vi "Write Tab-Delimited File.vi"() -> ()   [LabVIEW 2023]
doc: "Converts an array of data to a row of tab-separated columns, prepends the timestamp column, and terminates each row with the end of line character."
panel:
  out "Current Data":dbl[](graph)
  # "Overview: Demonstrates the use of the File I/O functions to write data to a tab-delimited text file.\nInstructions:\n1. Run this VI, which generates 5 sets of random data.\n2. Drag the [LabVIEW Data]\\Example Tab-Delimited File.txt file into a spreadsheet application like Microsoft Excel. The data in the file should be automatically populated in the spreadsheet.\n3. Close the spreadsheet application.\n4. Open Read Tab-Delimited File.vi and follow the instructions on its front panel to see an example of reading tab-delimited data in LabVIEW."
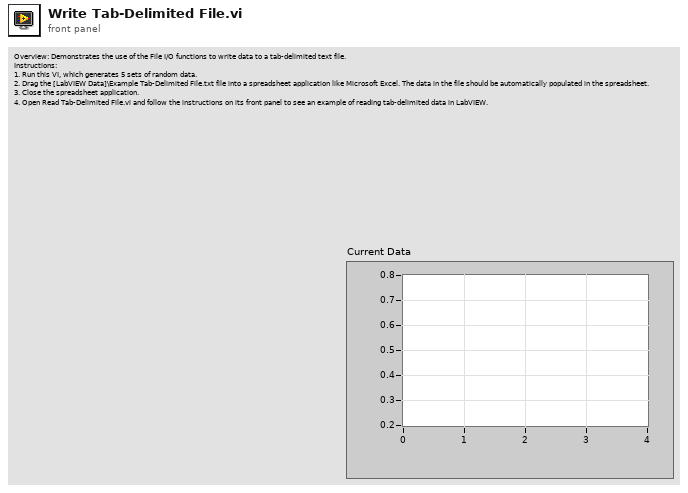
[diagram p1: front panel]
types:
  T1 = enum16{"open", "replace", "create", "open or create", "replace or create", "replace or create with confirmation"}
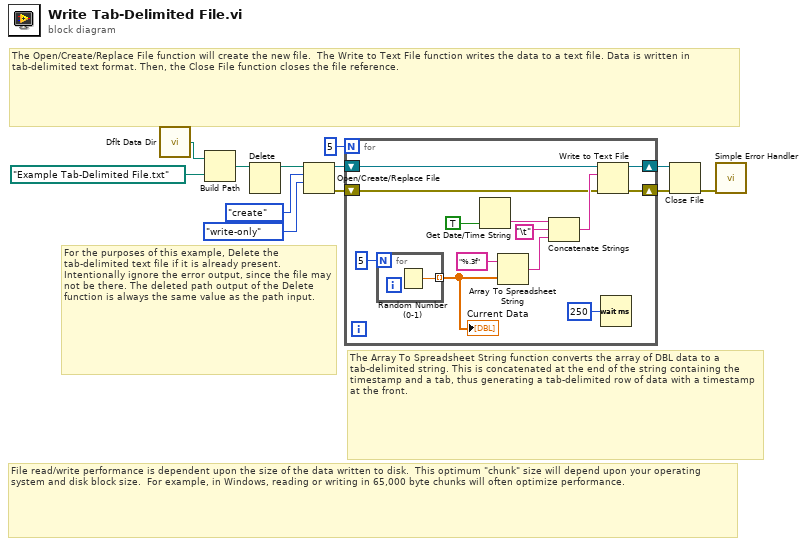
[diagram p0: block diagram]
diagram:
  # "File read/write performance is dependent upon the size of the data written to disk.  This optimum \"chunk\" size will depend upon your operating system and disk block size.  For example, in Windows, reading or writing in 65,000 byte chunks will often optimize performance."
  # "The Array To Spreadsheet String function converts the array of DBL data to a tab-delimited string. This is concatenated at the end of the string containing the timestamp and a tab, thus generating a tab-delimited row of data with a timestamp at the front."
  # "The Open/Create/Replace File function will create the new file.  The Write to Text File function writes the data to a text file. Data is written in tab-delimited text format. Then, the Close File function closes the file reference."
  # "For the purposes of this example, Delete the tab-delimited text file if it is already present. Intentionally ignore the error output, since the file may not be there. The deleted path output of the Delete function is always the same value as the path input."
  n1 = call <vilib>:"Dflt Data Dir.vi"() -> ("App:Default Data Directory"=w2:path)
  n2 = Build Path(base path=w2, name or relative path=path "Example Tab-Delimited File.txt" ("default name")) -> (appended path=w4:path)
  n3 = Delete(path (use dialog)=w4) -> (deleted path=w1:path)  [unwired: 4 in, 2 out]
  n4 = Open/Create/Replace File(file path (use dialog)=w1, operation (0:open)=T1."create", access (0:read/write)=enum16{"read/write", "read-only", "write-only"}."write-only") -> (refnum out=w9:refnum<file>, error out=w8:errorcluster)  [unwired: 1 in, 3 out]
  n5 = for {
    N: 5 ("number of acquisitions") -> [_]
    shift-right: [w22] -> w12
    shift-left: w9 -> [w20]
    shift-right: [w15] -> w11
    shift-left: w8 -> [w19]
    n6 = for {
      N: 5 ("number of points/acquisition") -> [_]
      tunnel: [w26] -> w17 mode=indexing
      n7 = Random Number (0-1)() -> (number: 0 to 1=w26:dbl)
    }
    "Current Data" <- w17
    n8 = Get Date/Time String(want seconds? (F)=TRUE) -> (time string=w16:string)  [unwired: 2 in, 1 out]
    n9 = Array To Spreadsheet String(array=w17, 3:"%.3f") -> (spreadsheet string=w24:string)  [unwired: 1 out]
    n10 = Concatenate Strings(w16, "\t" ("Tab"), w24) -> (w21:string)
    n11 = Write to Text File(file (use dialog)=w20, text=w21, error in=w19) -> (refnum out=w22:refnum<file>, error out=w15:errorcluster)  [unwired: 1 in, 1 out]
    n12 = Wait (ms)(milliseconds to wait=u32 250) -> ()  [unwired: 1 out]
  }
  n13 = Close File(refnum=w12, error in=w11) -> (error out=w10:errorcluster)  [unwired: 1 out]
  n14 = call <vilib>:"Simple Error Handler.vi"("error in (no error)"=w10) -> ()  [unwired: 1 in, 8 out]
